vi "Poll Controller.vi"(8 "error in (no error)":errorcluster, 11 "Filter Wheel in":refnum<class "Filter Wheel.lvclass">) -> (0 "error out":errorcluster, 2 "curr position":variant, 3 "Filter Wheel out":refnum<class "Filter Wheel.lvclass">)   [LabVIEW 2024, in "Filter Wheel.lvclass"]
uses:
  Filter Wheel.lvclass
  FW cluster Status.ctl
  FW enum status.ctl
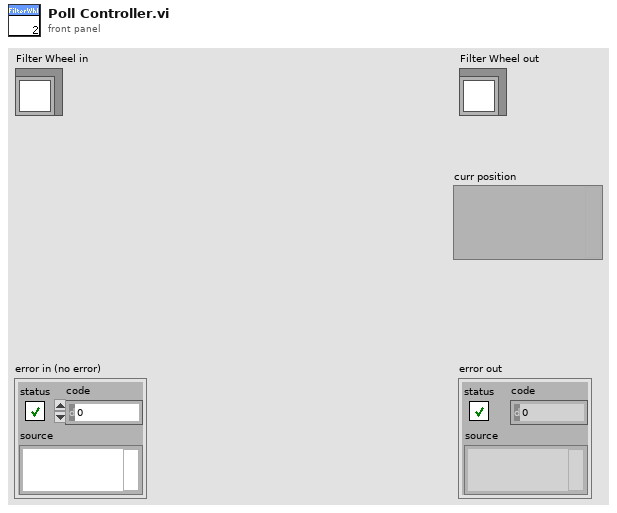
[diagram p1: front panel]
types:
  T1 = typedef "FW cluster Status.ctl" = cluster{"State":T2, "Positions":i32[], "Names":string[], "Notch":bool[], "Moving":bool[]}
  T2 = typedef "FW enum status.ctl" = enum16{"Initializing", "Moving", "Move Complete", "Error"}
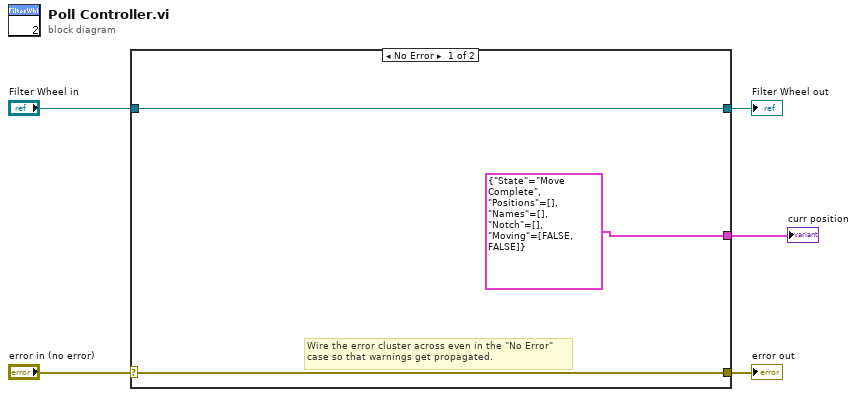
[diagram p0: block diagram]
diagram:
  n1 = case shown="No Error" "error in (no error)" {
    selector: "error in (no error)" -> [w7 w10]
    tunnel: [w7 w10] -> w4
    tunnel: [w8 w9] -> w2
    tunnel: "Filter Wheel in" -> [w8 w9]
    tunnel: [T1 {"State"=enum."Move Complete", "Positions"=[], "Names"=[], "Notch"=[], "Moving"=[FALSE, FALSE]} ("FW Status") _] -> w1
    frame No Error {
      # "Wire the error cluster across even in the \"No Error\"\ncase so that warnings get propagated."
    }
    frame Error {
    }
  }
  "error out" <- w4
  "Filter Wheel out" <- w2
  "curr position" <- w1
